vi "_Clear String - BD.vi"(0 "GObject in":refnum<vi>, 5 "error in (no error)":errorcluster) -> (14 "changed?":bool, 19 "error out":errorcluster)   [LabVIEW 2015, in "QD_Erease Data.lvlib"]
uses:
  QD_Erease Data.lvlib
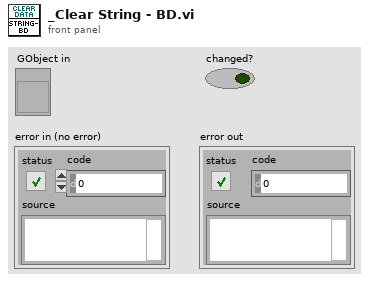
[diagram p1: front panel]
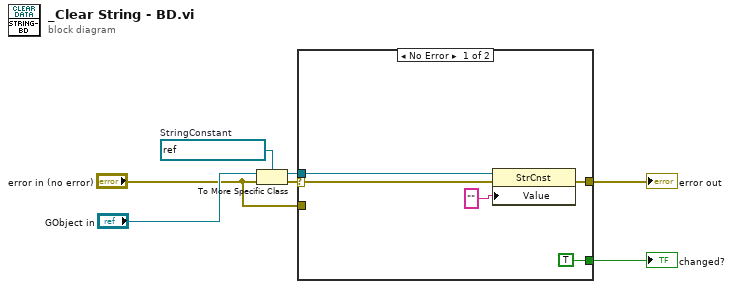
[diagram p0: block diagram]
diagram:
  w6 = refnum<vi> refnum  # StringConstant
  n1 = To More Specific Class(target class=w6, reference="GObject in", error in="error in (no error)") -> (specific class reference=w2:refnum<vi>, error out=w3:errorcluster)
  n2 = case shown="No Error" w3 {
    selector: w3 -> [w12 _]
    tunnel: [w10 w13] -> w1
    tunnel: w2 -> [w11 _]
    tunnel: "error in (no error)" -> [_ w13]
    tunnel: [TRUE _] -> w7
    frame No Error {
      n3 = property class="StrCnst"(reference=w11, error in=w12, "Value"="") -> (error out=w10:errorcluster)  [unwired: 1 out]
    }
    frame Error {
    }
  }
  "changed?" <- w7
  "error out" <- w1
